vi "GEOM_CheckMixedROIs.vi"(9 "roi coord2":T1, 10 "roi coord1":T1) -> (1 "y mixed":bool, 2 "x mixed":bool, 3 "mixed":bool)   [LabVIEW 2016]
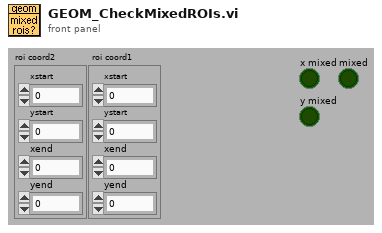
[diagram p1: front panel]
types:
  T1 = cluster{"xstart":i32, "ystart":i32, "xend":i32, "yend":i32}
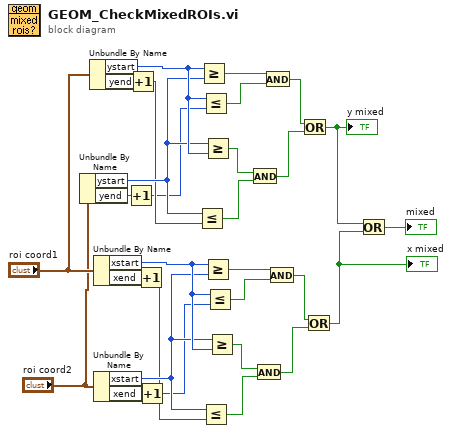
[diagram p0: block diagram]
diagram:
  n1 = Unbundle By Name("roi coord2") -> ("ystart"=w17:i32, "yend"=w20:i32)
  n2 = Unbundle By Name("roi coord1") -> ("ystart"=w18:i32, "yend"=w16:i32)
  n3 = Unbundle By Name("roi coord1") -> ("xstart"=w27:i32, "xend"=w5:i32)
  n4 = Unbundle By Name("roi coord2") -> ("xstart"=w26:i32, "xend"=w6:i32)
  n5 = Increment(x=w20) -> (x+1=w1:i32)
  n6 = Increment(x=w16) -> (x+1=w2:i32)
  n7 = Increment(x=w5) -> (x+1=w3:i32)
  n8 = Increment(x=w6) -> (x+1=w4:i32)
  n9 = Less Or Equal?(x=w17, y=w2) -> (x <= y?=w14:bool)
  n10 = Greater Or Equal?(x=w18, y=w17) -> (x >= y?=w21:bool)
  n11 = Less Or Equal?(x=w18, y=w1) -> (x <= y?=w19:bool)
  n12 = Less Or Equal?(x=w26, y=w3) -> (x <= y?=w24:bool)
  n13 = Greater Or Equal?(x=w17, y=w18) -> (x >= y?=w15:bool)
  n14 = Greater Or Equal?(x=w27, y=w26) -> (x >= y?=w29:bool)
  n15 = Less Or Equal?(x=w27, y=w4) -> (x <= y?=w28:bool)
  n16 = Greater Or Equal?(x=w26, y=w27) -> (x >= y?=w25:bool)
  n17 = And(x=w15, y=w14) -> (x .and. y?=w12:bool)
  n18 = And(x=w25, y=w24) -> (x .and. y?=w22:bool)
  n19 = And(x=w21, y=w19) -> (x .and. y?=w13:bool)
  n20 = And(x=w29, y=w28) -> (x .and. y?=w23:bool)
  n21 = Or(x=w13, y=w12) -> (x .or. y?=w9:bool)
  "y mixed" <- w9
  n22 = Or(x=w23, y=w22) -> (x .or. y?=w7:bool)
  "x mixed" <- w7
  n23 = Or(x=w9, y=w7) -> (x .or. y?=→"mixed":bool)
